vi "IR_OPO_esp_gpib_init_system.vi"(1 "Device In":u8=1) -> (0 "Device Out":u8)   [LabVIEW 2015]
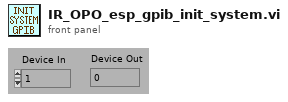
[diagram p1: front panel]
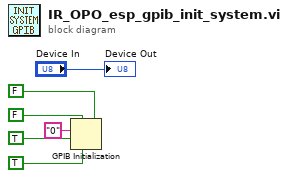
[diagram p0: block diagram]
diagram:
  n1 = GPIB Initialization(1:FALSE, 2:TRUE, 3:FALSE ("assert REN with IFC (T)"), 5:TRUE ("IST bit sense (T)"), 6:"0" ("address string")) -> ()  [unwired: 2 in, 1 out]
  "Device Out" <- "Device In"
